vi "Read Write Sample Code - JKI SM.vi"(8 "error in (no error)":errorcluster) -> (0 "error out":errorcluster)   [LabVIEW 2020]
panel:
  in  "stop":bool
  in  "讀取目標字數":i32=1
  in  "Write":bool
  in  "VISA resource name":refnum<visa-resource-name>
  out "read buffer":string
  in  "write buffer":string
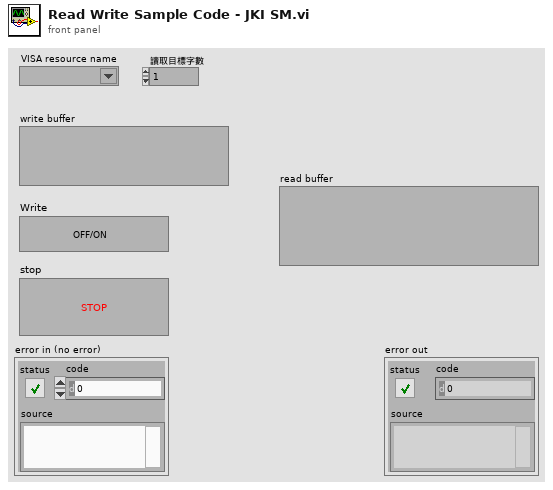
[diagram p1: front panel]
types:
  T1 = enum32{"Invalid", "Standard", "Closed", "Hidden", "Minimized", "Maximized"}
  T2 = enum32{"invalid app kind", "Development System", "Run Time System", "Student Edition", "Embedded LabVIEW", "Evaluation", "Custom"}
  T3 = cluster{"Core":cluster{"Current VI Reference":refnum<vi>, "Close Panel on Exit?":bool}, "VISA resource name":refnum<visa-resource-name>, "Serial Settings:Number of Bytes at Serial Port":u32, "read buffer":string}
  T4 = cluster{"Current VI Reference":refnum<vi>, "Close Panel on Exit?":bool}
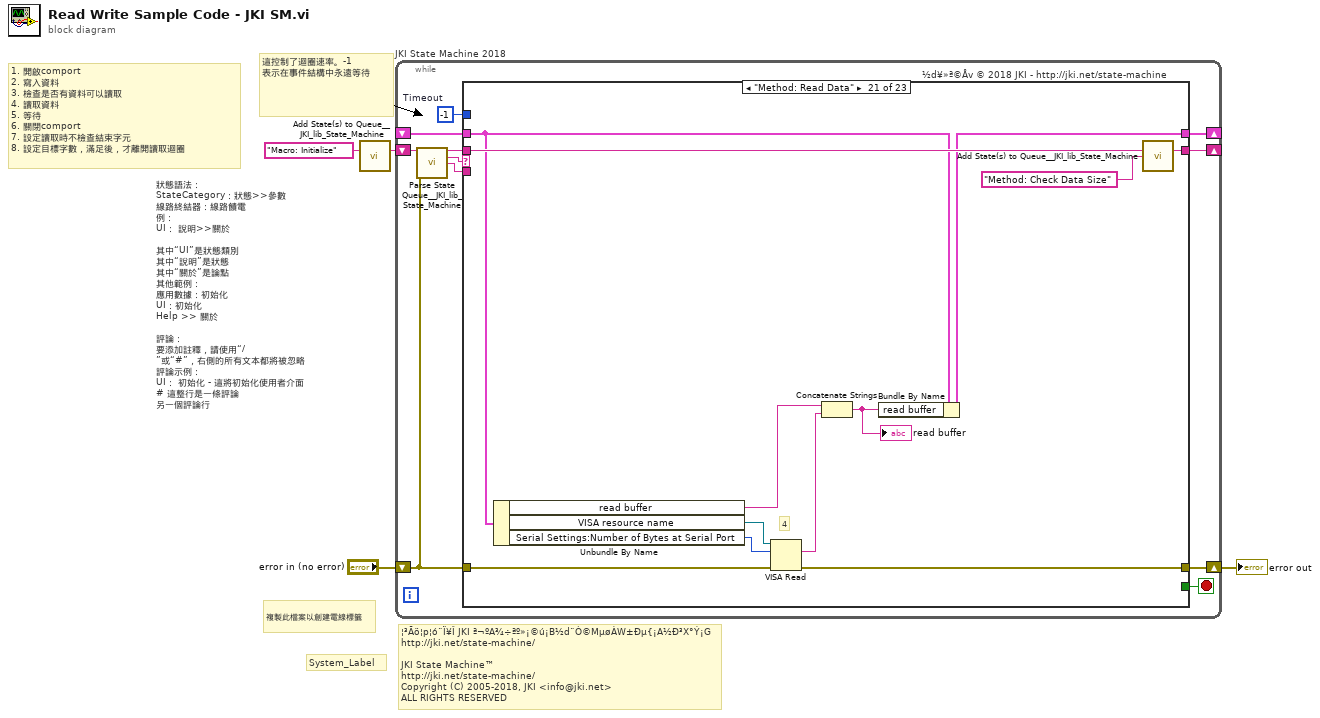
[diagram p0: block diagram]
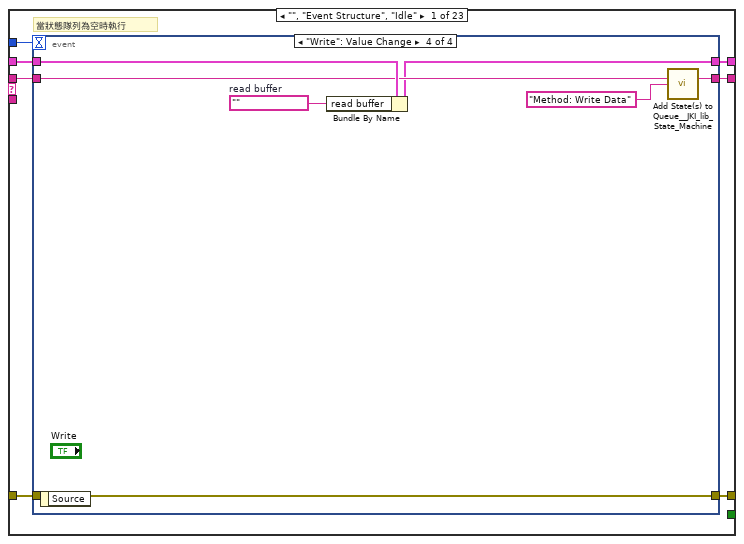
[diagram p2: hidden frame]
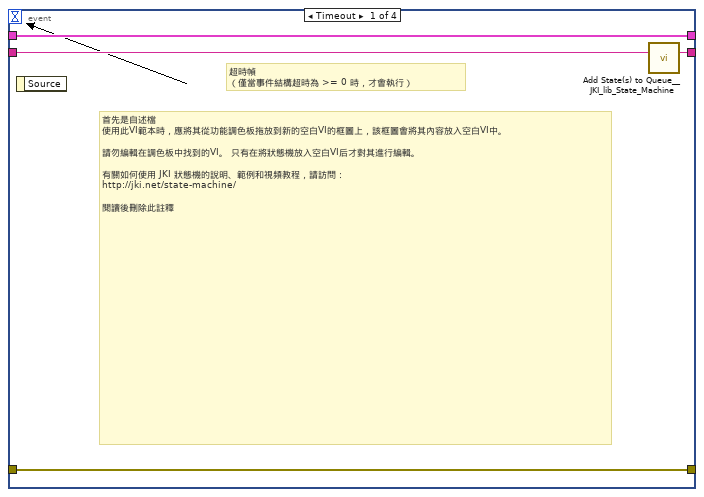
[diagram p3: hidden frame]
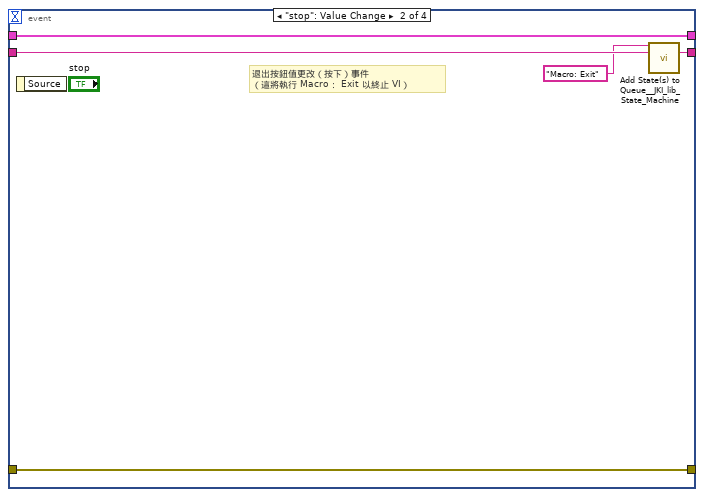
[diagram p4: hidden frame]
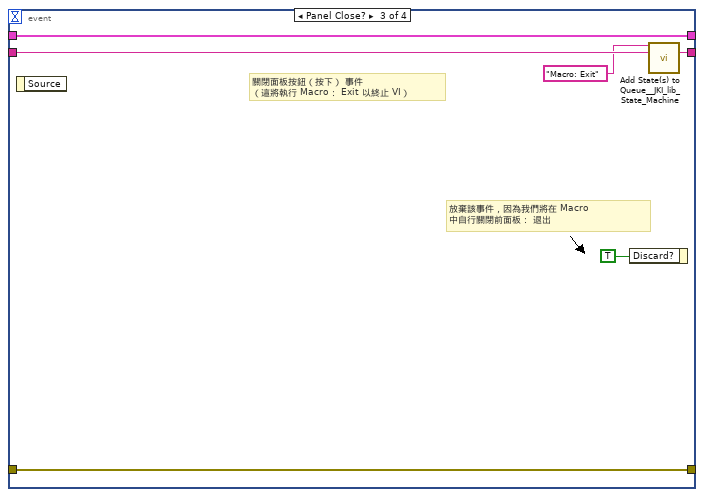
[diagram p5: hidden frame]
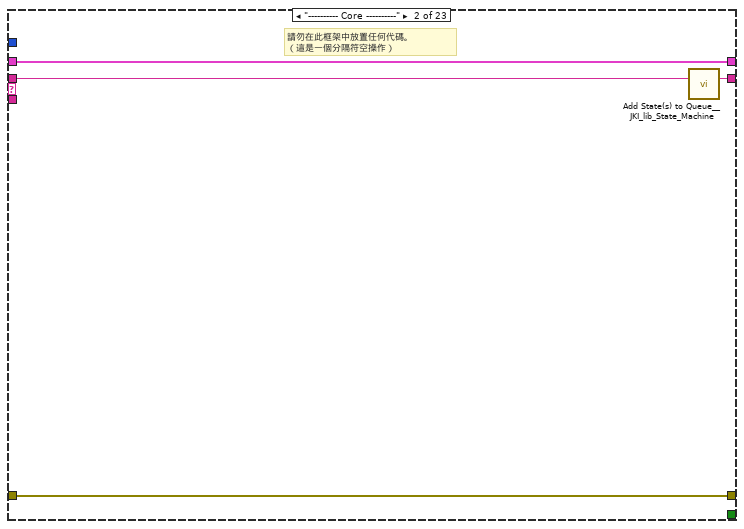
[diagram p6: hidden frame]
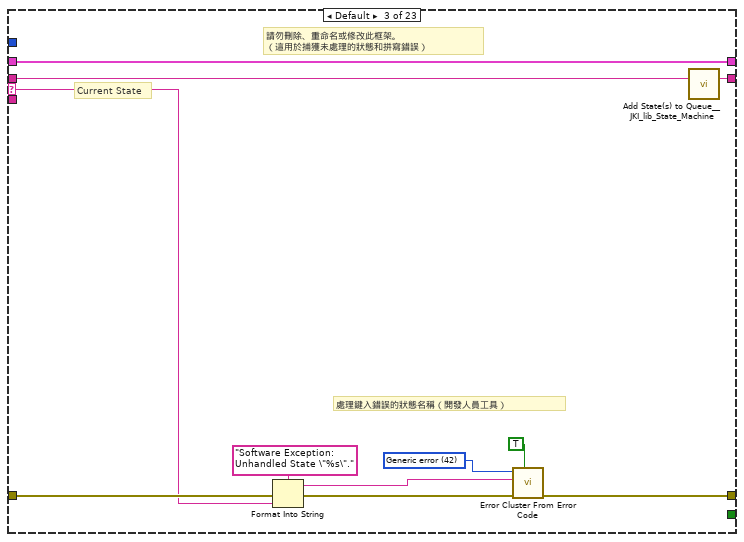
[diagram p7: hidden frame]
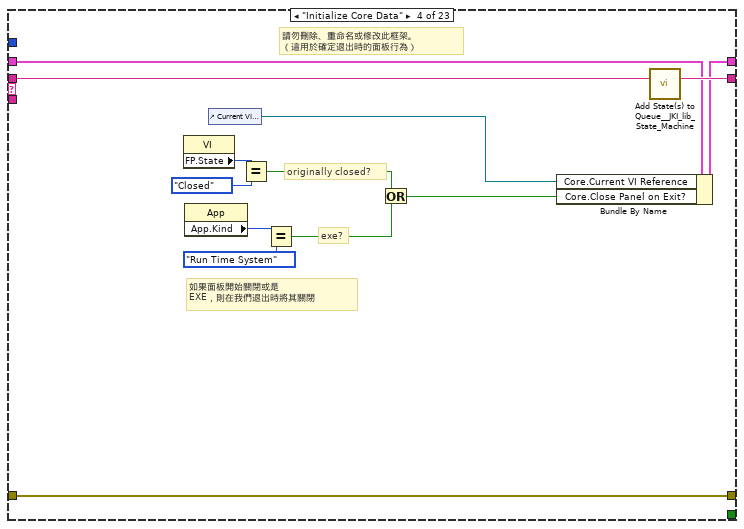
[diagram p8: hidden frame]
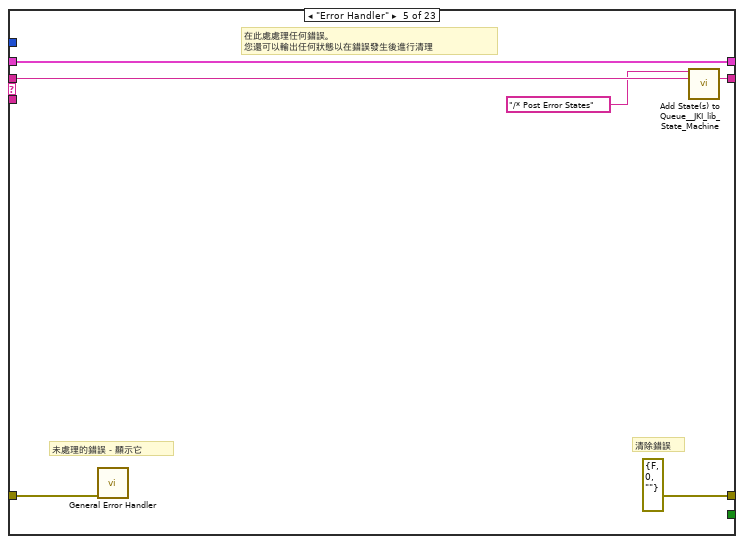
[diagram p9: hidden frame]
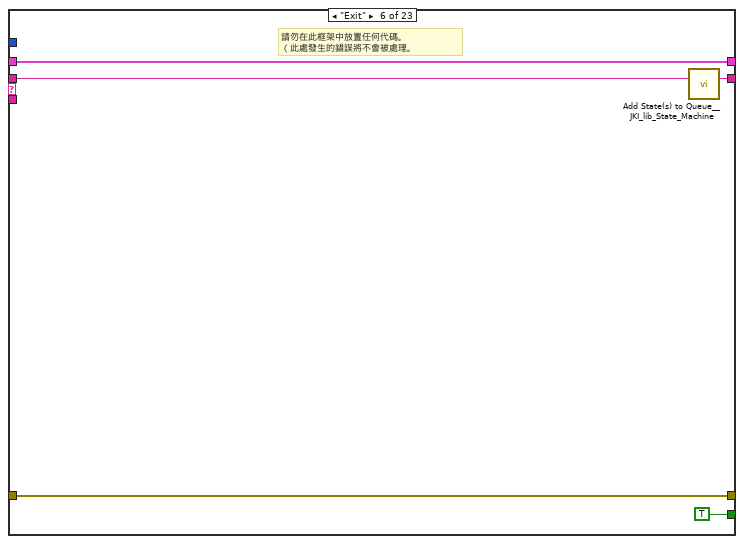
[diagram p10: hidden frame]
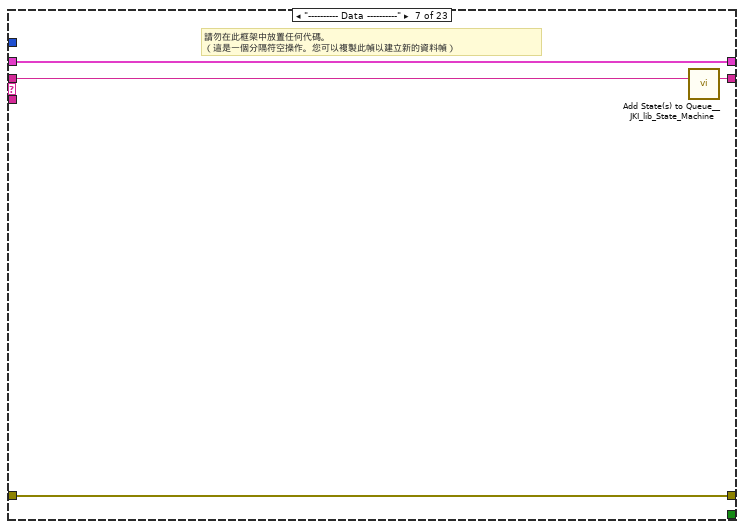
[diagram p11: hidden frame]
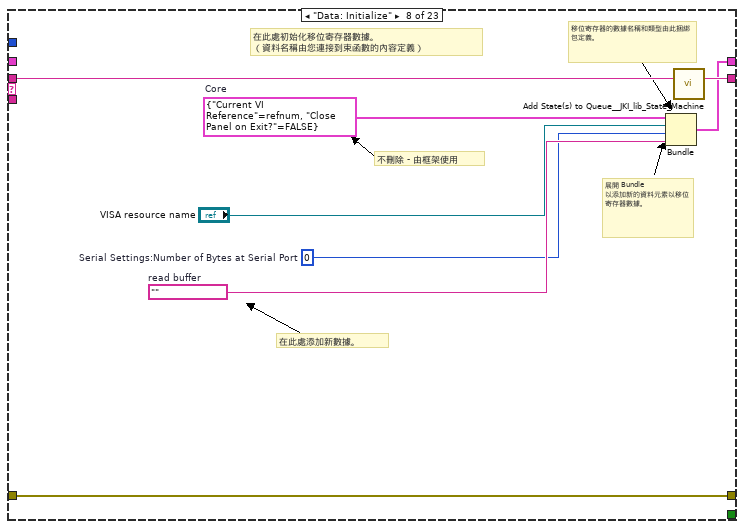
[diagram p12: hidden frame]
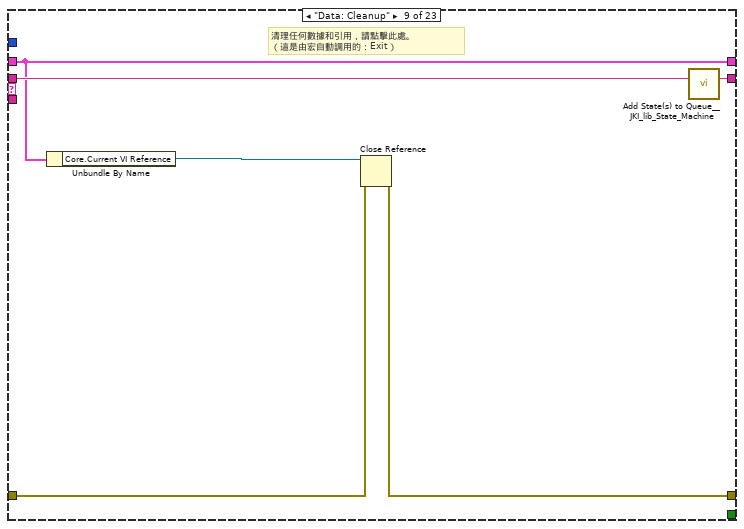
[diagram p13: hidden frame]
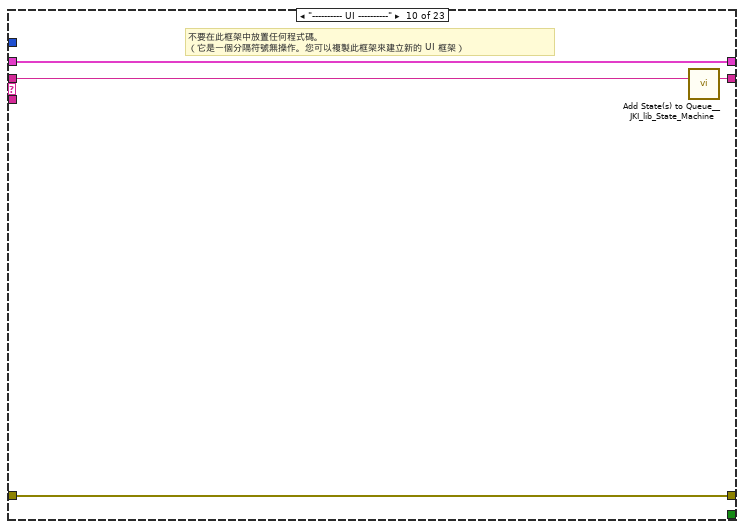
[diagram p14: hidden frame]
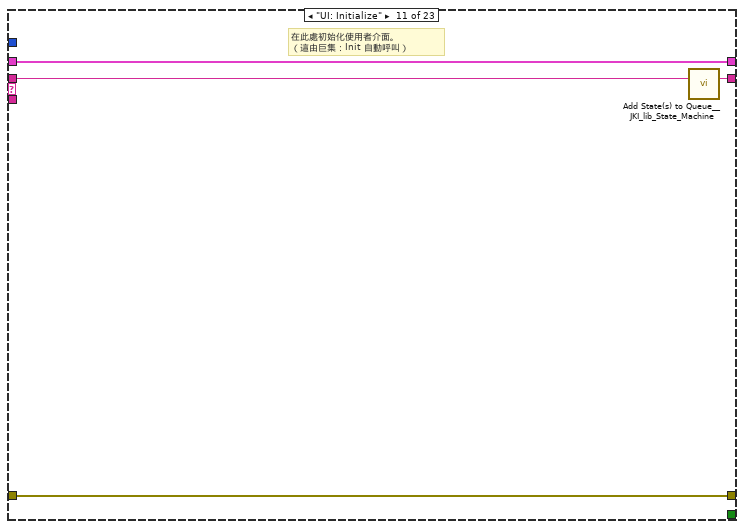
[diagram p15: hidden frame]
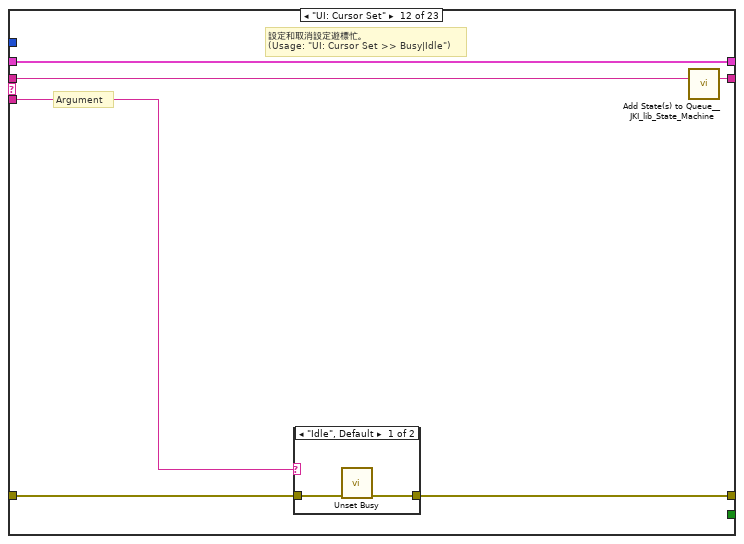
[diagram p16: hidden frame]
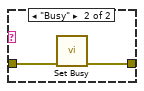
[diagram p17: hidden frame]
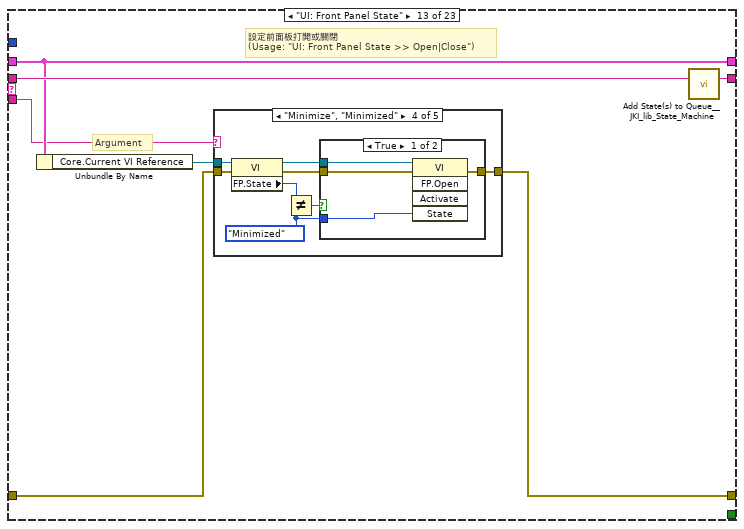
[diagram p18: hidden frame]
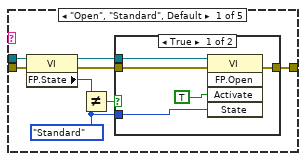
[diagram p19: hidden frame]
diagram:
  # "¦³Ãö¦p¦ó¨Ï¥Î JKI ª¬ºA¾÷ªº»¡©ú¡B½d¨Ò©MµøÀW±Ðµ{¡A½Ð³X°Ý¡G\nhttp://jki.net/state-machine/\n\nJKI State Machine™\nhttp://jki.net/state-machine/\nCopyright (C) 2005-2018, JKI <info@jki.net>\nALL RIGHTS RESERVED"
  # "狀態語法：\nStateCategory：狀態>>參數\n線路終結器：線路饋電\n例：\nUI： 說明>>關於\n\n其中“UI”是狀態類別\n其中“說明”是狀態\n其中“關於”是論點\n其他範例：\n應用數據：初始化\nUI：初始化\nHelp >> 關於\n\n評論：\n要添加註釋，請使用“/”或“#”，右側的所有文本都將被忽略\n評論示例：\nUI： 初始化 - 這將初始化使用者介面\n# 這整行是一條評論\n另一個評論行"
  # "複製此檔案以創建電線標籤"
  # "這控制了迴圈速率。-1 表示在事件結構中永遠等待"
  # "System_Label"
  # "1. 開啟comport\n2. 寫入資料\n3. 檢查是否有資料可以讀取\n4. 讀取資料\n5. 等待\n6. 關閉comport\n7. 設定讀取時不檢查結束字元\n8. 設定目標字數，滿足後，才離開讀取迴圈"
  n1 = call <vilib>:"Add State(s) to Queue__JKI_lib_State_Machine.vi"("State(s) in (\"\")"="Macro: Initialize") -> ("States Out"=w4:string)  [unwired: 14 in]
  n2 = while "JKI State Machine 2018" {
    shift-right: [w8] -> _
    shift-left: _ -> [w7]
    shift-right: [w11] -> w1
    shift-left: "error in (no error)" -> [w5]
    shift-right: [w10] -> _
    shift-left: w4 -> [w12]
    stop <- w9 stop-if-true
    w6 = -1  # Timeout
    # "½d¥»ª©Åv © 2018 JKI - http://jki.net/state-machine"
    n3 = call <vilib>:"Parse State Queue__JKI_lib_State_Machine.vi"("State Queue"=w12, "Error In (no error)"=w5) -> ("Remaining States"=w14:string, "Current State"=w15:string, "Arguments"=w13:string)  [unwired: 11 in]
    n4 = case shown="\"Method: Read Data\"" w15 {
      selector: w15 -> [_ _ w49 _ _ _ _ _ _ _ _ _ _ _ _ _ _ _ _ _ _ _ _]
      tunnel: w14 -> [w22 w48 w53 w72 w78 w83 w87 w95 w101 w105 w109 w115 w126 w195 w200 w210 w214 w220 w233 w241 w253 w264 w272]
      tunnel: w13 -> [_ _ _ _ _ _ _ _ _ _ _ w110 w120 _ _ _ _ _ _ _ _ _ _]
      tunnel: w7 -> [w20 w45 w51 w65 w75 w81 w84 _ w96 w102 w107 w113 w122 w192 w197 w207 w211 w215 w231 w235 w249 w259 w268]
      tunnel: [w19 w46 w55 w69 errorcluster {"status"=FALSE, "code"=0, "source"=""} ("error out") w80 w85 w92 w97 w103 w106 w111 w123 w193 w198 w208 w212 w217 w230 w237 w251 w262 w270] -> w11
      tunnel: w5 -> [w18 w46 w54 w69 w74 w80 w85 w92 w98 w103 w106 w112 w124 w193 w198 w208 w212 w218 w229 w236 w250 w262 w269]
      tunnel: [w21 w47 w52 w71 w77 w82 w86 w94 w100 w104 w108 w114 w125 w194 w199 w209 w213 w219 w232 w240 w252 w263 w271] -> w10
      tunnel: [_ _ _ _ _ TRUE _ _ _ _ _ _ _ _ _ _ _ _ _ _ _ _ _] -> w9
      tunnel: [w17 w45 w51 w70 w75 w81 w84 w93 w96 w102 w107 w113 w122 w192 w197 w207 w211 w216 w231 w235 w246 w259 w268] -> w8
      tunnel: w6 -> [w16 _ _ _ _ _ _ _ _ _ _ _ _ _ _ _ _ _ _ _ _ _ _]
      frame "", "Event Structure", "Idle" {
        # "當狀態隊列為空時執行"
        n5 = event shown="[3] \"Write\": Value Change" {
          selector: _ -> [_ _ _ _]
          dyn-events: _ -> [_ _ _ _]
          timeout: w16 -> [_ _ _ _]
          tunnel: w22 -> [w26 w31 w37 w41]
          tunnel: [w25 w30 w36 w42] -> w21
          tunnel: w20 -> [w23 w28 w34 w44]
          tunnel: [w24 w29 w35 w43] -> w19
          tunnel: w18 -> [w24 w29 w35 w43]
          tunnel: [w23 w28 w34 w40] -> w17
          event Timeout {
            # "首先是自述檔\n使用此VI範本時，應將其從功能調色板拖放到新的空白VI的框圖上，該框圖會將其內容放入空白VI中。\n\n請勿編輯在調色板中找到的VI。 只有在將狀態機放入空白VI后才對其進行編輯。\n\n有關如何使用 JKI 狀態機的說明、範例和視頻教程，請訪問：\nhttp://jki.net/state-machine/\n\n閱讀後刪除此註釋"
            # "超時幀\n（僅當事件結構超時為 >= 0 時，才會執行）"
            n6 = event-data() -> ()  [unwired: 1 in, 1 out]
            n7 = call <vilib>:"Add State(s) to Queue__JKI_lib_State_Machine.vi"("State(s) in (\"\")"=w26) -> ("States Out"=w25:string)  [unwired: 14 in]
          }
          event "stop": Value Change {
            # "退出按鈕值更改（按下）事件\n（這將執行 Macro： Exit 以終止 VI）"
            n8 = event-data() -> ()  [unwired: 1 in, 1 out]
            n9 = call <vilib>:"Add State(s) to Queue__JKI_lib_State_Machine.vi"("State(s) in Front (\"\")"="Macro: Exit", "State(s) in (\"\")"=w31) -> ("States Out"=w30:string)  [unwired: 13 in]
          }
          event Panel Close? {
            # "放棄該事件，因為我們將在 Macro 中自行關閉前面板： 退出"
            # "關閉面板按鈕（按下） 事件\n（這將執行 Macro： Exit 以終止 VI）"
            n10 = event-data() -> ()  [unwired: 1 in, 1 out]
            n11 = event-data("Discard?"=TRUE) -> ()  [unwired: 1 in, 1 out]
            n12 = call <vilib>:"Add State(s) to Queue__JKI_lib_State_Machine.vi"("State(s) in Front (\"\")"="Macro: Exit", "State(s) in (\"\")"=w37) -> ("States Out"=w36:string)  [unwired: 13 in]
          }
          event "Write": Value Change {
            w39 = ""  # read buffer
            n13 = event-data() -> ()  [unwired: 1 in, 1 out]
            n14 = Bundle By Name(cluster=w44, "read buffer"=w39) -> (w40:T3)
            n15 = call <vilib>:"Add State(s) to Queue__JKI_lib_State_Machine.vi"("State(s) in (\"\")"=w41, "State(s) at Back (\"\")"="Method: Write Data" ("State(s) at Back (\"\")")) -> ("States Out"=w42:string)  [unwired: 13 in]
          }
        }
      }
      frame "---------- Core ----------" {
        # "請勿在此框架中放置任何代碼。\n（這是一個分隔符空操作）"
        n16 = call <vilib>:"Add State(s) to Queue__JKI_lib_State_Machine.vi"("State(s) in (\"\")"=w48) -> ("States Out"=w47:string)  [unwired: 14 in]
      }
      frame Default {
        w58 = 42 items=["No error", "Argument error", "Memory is full", "Out of zone", "End of file", "File already open", "Generic file I/O error", "File not found", "File permission error", "Disk is full", "Duplicate path", "Too many files open", "System feature not enabled", "Resource file not found", "Cannot add resource", "Resource not found", "Image not found", "Image memory error", "Pen does not exist", "Config type invalid", "Config token not found", "Config parse error", "Config memory error", "Bad external code format", "Bad external code offset", "External code not present", "Null window", "Destroy window error", "Null menu", "Print aborted", "Bad print record", "Print driver error", "Windows error during printing", "Memory error during printing", "Print dialog error", "Generic print error", "Invalid device refnum", "Device not found", "Device parameter error", "Device unit error", "Cannot open device", "Device call aborted", "Generic error", "Cancelled by user", "Object ID too low", "Object ID too high", "Object not in heap", "Unknown heap", "Unknown object (invalid DefProc)", "Unknown object (DefProc not in table)", "Message out of range", "Invalid (null) method", "Unknown message", "Manager call not supported", "Bad address", "Network operation in progress", "Network operation timed out", "Connection is busy", "Network attribute not supported", "Network error", "Address in use", "System out of memory", "Connection aborted", "Connection refused", "Not connected", "Already connected", "Connection closed", "Initialization error (interapplication manager)", "Bad occurrence", "Wait on unbound occurrence handler", "Occurrence queue overflow", "Datalog type conflict", "Unused", "Unrecognized type (interapplication manager)", "Memory corrupt", "Failed to make temporary DLL", "Old CIN version", "Drag socket not found", "Failed to load drop-object", "Failed to register OLE object", "Failed to release OLE object", "Format specifier type mismatch", "Unknown format specifier", "Too few format specifiers", "Too many format specifiers", "Scan failed", "Newer CIN version", "Error converting to variant", "Runtime menu error", "Password tampered", "Variant attribute not found", "Incompatible variant data type", "Event data is not available", "Event Store is not present", "Occurrence is not found", "Event Queue is not created", "Event info is not available", "Refnum passed is NULL", "Error retrieving Class GUID", "Error retrieving CoClass GUID", "Error retrieving TypeLib GUID.", "Bad built application magic bytes.", "Specific driver is different from the specific driver associated with the Logical Name.", "There is no session opened to the class driver.", "Max Error", "MAX - Error with config objects", "MAX - Error loading configuration", "MAX - Group not supported"]
        # "Current State"
        # "請勿刪除、重命名或修改此框架。\n（這用於捕獲未處理的狀態和拼寫錯誤）"
        # "處理鍵入錯誤的狀態名稱（開發人員工具）"
        n17 = Format Into String(format string="Software Exception: Unhandled State \"%s\"." ("message"), error in=w54, w49) -> (resulting string=w57:string, error out=w56:errorcluster)  [unwired: 1 in]
        n18 = call <vilib>:"Error Cluster From Error Code.vi"("show call chain? (False)"=TRUE, "error in (no error)"=w56, "error message (\"\")"=w57, "error code (0)"=w58) -> ("error out"=w55:errorcluster)  [unwired: 5 in]
        n19 = call <vilib>:"Add State(s) to Queue__JKI_lib_State_Machine.vi"("State(s) in (\"\")"=w53) -> ("States Out"=w52:string)  [unwired: 14 in]
      }
      frame "Initialize Core Data" {
        # "請勿刪除、重命名或修改此框架。\n（這用於確定退出時的面板行為）"
        # "originally closed?"
        # "exe?"
        # "如果面板開始關閉或是 EXE，則在我們退出時將其關閉"
        n20 = property class="VI"() -> ("FP.State"=w62:T1)  [unwired: 2 in, 2 out]
        n21 = property class="App"() -> ("App.Kind"=w68:T2)  [unwired: 2 in, 2 out]
        n22 = control-ref of="Current VI Reference"() -> (w63:refnum<vi>)
        n23 = Equal?(x=w62, y=T1."Closed" ("Front Panel Window:State")) -> (x = y?=w60:bool)
        n24 = Equal?(x=w68, y=T2."Run Time System" ("Application:Kind")) -> (x = y?=w66:bool)
        n25 = Or(x=w60, y=w66) -> (x .or. y?=w64:bool)
        n26 = Bundle By Name(cluster=w65, "Core.Current VI Reference"=w63, "Core.Close Panel on Exit?"=w64) -> (w70:T3)
        n27 = call <vilib>:"Add State(s) to Queue__JKI_lib_State_Machine.vi"("State(s) in (\"\")"=w72) -> ("States Out"=w71:string)  [unwired: 14 in]
      }
      frame "Error Handler" {
        # "未處理的錯誤－顯示它"
        # "在此處處理任何錯誤。\n您還可以輸出任何狀態以在錯誤發生後進行清理"
        # "清除錯誤"
        n28 = call <vilib>:"General Error Handler.vi"("error in (no error)"=w74) -> ()  [unwired: 10 in, 5 out]
        n29 = call <vilib>:"Add State(s) to Queue__JKI_lib_State_Machine.vi"("State(s) in Front (\"\")"="/* Post Error States", "State(s) in (\"\")"=w78) -> ("States Out"=w77:string)  [unwired: 13 in]
      }
      frame "Exit" {
        # "請勿在此框架中放置任何代碼。\n（此處發生的錯誤將不會被處理。"
        n30 = call <vilib>:"Add State(s) to Queue__JKI_lib_State_Machine.vi"("State(s) in (\"\")"=w83) -> ("States Out"=w82:string)  [unwired: 14 in]
      }
      frame "---------- Data ----------" {
        # "請勿在此框架中放置任何代碼。\n（這是一個分隔符空操作。您可以複製此幀以建立新的資料幀）"
        n31 = call <vilib>:"Add State(s) to Queue__JKI_lib_State_Machine.vi"("State(s) in (\"\")"=w87) -> ("States Out"=w86:string)  [unwired: 14 in]
      }
      frame "Data: Initialize" {
        w88 = u32 0  # Serial Settings:Number of Bytes at Serial Port
        w90 = T4 {"Current VI Reference"=refnum, "Close Panel on Exit?"=FALSE}  # Core
        w91 = ""  # read buffer
        # "不刪除 - 由框架使用"
        # "展開 Bundle 以添加新的資料元素以移位寄存器數據。"
        # "在此處添加新數據。"
        # "移位寄存器的數據名稱和類型由此捆綁包定義。"
        # "在此處初始化移位寄存器數據。\n（資料名稱由您連接到束函數的內容定義）"
        n32 = Bundle("Core"=w90, "VISA resource name"="VISA resource name", "Serial Settings:Number of Bytes at Serial Port"=w88, "read buffer"=w91) -> (w93:T3)  [unwired: 1 in]
        n33 = call <vilib>:"Add State(s) to Queue__JKI_lib_State_Machine.vi"("State(s) in (\"\")"=w95) -> ("States Out"=w94:string)  [unwired: 14 in]
      }
      frame "Data: Cleanup" {
        # "清理任何數據和引用，請點擊此處。\n（這是由宏自動調用的：Exit）"
        n34 = Unbundle By Name(w96) -> ("Core.Current VI Reference"=w99:refnum<vi>)
        n35 = Close Reference(reference=w99, error in (no error)=w98) -> (error out=w97:errorcluster)
        n36 = call <vilib>:"Add State(s) to Queue__JKI_lib_State_Machine.vi"("State(s) in (\"\")"=w101) -> ("States Out"=w100:string)  [unwired: 14 in]
      }
      frame "---------- UI ----------" {
        # "不要在此框架中放置任何程式碼。\n（它是一個分隔符號無操作。您可以複製此框架來建立新的 UI 框架）"
        n37 = call <vilib>:"Add State(s) to Queue__JKI_lib_State_Machine.vi"("State(s) in (\"\")"=w105) -> ("States Out"=w104:string)  [unwired: 14 in]
      }
      frame "UI: Initialize" {
        # "在此處初始化使用者介面。\n（這由巨集：Init 自動呼叫）"
        n38 = call <vilib>:"Add State(s) to Queue__JKI_lib_State_Machine.vi"("State(s) in (\"\")"=w109) -> ("States Out"=w108:string)  [unwired: 14 in]
      }
      frame "UI: Cursor Set" {
        # "Argument"
        # "設定和取消設定遊標忙。\n(Usage: \"UI: Cursor Set >> Busy|Idle\")"
        n39 = case shown="\"Idle\", Default" w110 {
          tunnel: w112 -> [w117 w119]
          tunnel: [w116 w118] -> w111
          frame "Idle", Default {
            n40 = call <vilib>:"Unset Busy.vi"("error in (no error)"=w117) -> ("error out"=w116:errorcluster)  [unwired: 10 in]
          }
          frame "Busy" {
            n41 = call <vilib>:"Set Busy.vi"("error in (no error)"=w119) -> ("error out"=w118:errorcluster)  [unwired: 9 in, 1 out]
          }
        }
        n42 = call <vilib>:"Add State(s) to Queue__JKI_lib_State_Machine.vi"("State(s) in (\"\")"=w115) -> ("States Out"=w114:string)  [unwired: 14 in]
      }
      frame "UI: Front Panel State" {
        # "Argument"
        # "設定前面板打開或關閉\n(Usage: \"UI: Front Panel State >> Open|Close\")"
        n43 = Unbundle By Name(w122) -> ("Core.Current VI Reference"=w121:refnum<vi>)
        n44 = case shown="\"Minimize\", \"Minimized\"" w120 {
          tunnel: w124 -> [w132 w147 w158 w171 w184]
          tunnel: [w134 w148 w160 w173 w186] -> w123
          tunnel: w121 -> [w133 w145 w159 w172 w185]
          frame "Open", "Standard", Default {
            w127 = T1."Standard" ("State")
            n45 = property class="VI"(reference=w133, error in=w132) -> (reference out=w130:refnum<vi>, error out=w131:errorcluster, "FP.State"=w129:T1)
            n46 = Not Equal?(x=w129, y=w127) -> (x != y?=w128:bool)
            n47 = case shown="True" w128 {
              tunnel: [w138 w140] -> w134
              tunnel: w131 -> [w137 w140]
              tunnel: w130 -> [w136 _]
              tunnel: w127 -> [w135 _]
              frame True {
                n48 = invoke class="VI" method="FP.Open"(reference=w136, error in=w137, "Activate"=TRUE, "State"=w135) -> (error out=w138:errorcluster)  [unwired: 1 in, 4 out]
              }
              frame False {
              }
            }
          }
          frame "Close", "Closed" {
            n49 = property class="VI"(reference=w145, error in=w147) -> (reference out=w144:refnum<vi>, error out=w146:errorcluster, "FP.State"=w142:T1)
            n50 = Not Equal?(x=w142, y=T1."Closed" ("Front Panel Window:State")) -> (x != y?=w141:bool)
            n51 = case shown="True" w141 {
              tunnel: [w149 w152] -> w148
              tunnel: w146 -> [w149 w151]
              tunnel: w144 -> [_ w150]
              frame False {
              }
              frame True {
                n52 = invoke class="VI" method="FP.Close"(reference=w150, error in=w151) -> (error out=w152:errorcluster)  [unwired: 1 in, 2 out]
              }
            }
          }
          frame "Hidden", "Hide" {
            w153 = T1."Hidden" ("State")
            n53 = property class="VI"(reference=w159, error in=w158) -> (reference out=w156:refnum<vi>, error out=w157:errorcluster, "FP.State"=w155:T1)
            n54 = Not Equal?(x=w155, y=w153) -> (x != y?=w154:bool)
            n55 = case shown="True" w154 {
              tunnel: [w164 w165] -> w160
              tunnel: w157 -> [w163 w165]
              tunnel: w156 -> [w162 _]
              tunnel: w153 -> [w161 _]
              frame True {
                n56 = invoke class="VI" method="FP.Open"(reference=w162, error in=w163, "State"=w161) -> (error out=w164:errorcluster)  [unwired: 2 in, 4 out]
              }
              frame False {
              }
            }
          }
          frame "Minimize", "Minimized" {
            w166 = T1."Minimized" ("State")
            n57 = property class="VI"(reference=w172, error in=w171) -> (reference out=w169:refnum<vi>, error out=w170:errorcluster, "FP.State"=w168:T1)
            n58 = Not Equal?(x=w168, y=w166) -> (x != y?=w167:bool)
            n59 = case shown="True" w167 {
              tunnel: [w177 w178] -> w173
              tunnel: w170 -> [w176 w178]
              tunnel: w169 -> [w175 _]
              tunnel: w166 -> [w174 _]
              frame True {
                n60 = invoke class="VI" method="FP.Open"(reference=w175, error in=w176, "State"=w174) -> (error out=w177:errorcluster)  [unwired: 2 in, 4 out]
              }
              frame False {
              }
            }
          }
          frame "Maximize", "Maximized" {
            w179 = T1."Maximized" ("State")
            n61 = property class="VI"(reference=w185, error in=w184) -> (reference out=w182:refnum<vi>, error out=w183:errorcluster, "FP.State"=w181:T1)
            n62 = Not Equal?(x=w181, y=w179) -> (x != y?=w180:bool)
            n63 = case shown="True" w180 {
              tunnel: [w190 w191] -> w186
              tunnel: w183 -> [w189 w191]
              tunnel: w182 -> [w188 _]
              tunnel: w179 -> [w187 _]
              frame True {
                n64 = invoke class="VI" method="FP.Open"(reference=w188, error in=w189, "State"=w187) -> (error out=w190:errorcluster)  [unwired: 2 in, 4 out]
              }
              frame False {
              }
            }
          }
        }
        n65 = call <vilib>:"Add State(s) to Queue__JKI_lib_State_Machine.vi"("State(s) in (\"\")"=w126) -> ("States Out"=w125:string)  [unwired: 14 in]
      }
      frame "---------- Macro ----------" {
        # "不要在此框架中放置任何程式碼。\n（它是一個分隔符無操作。您可以複製該幀以創建新的巨集幀）"
        n66 = call <vilib>:"Add State(s) to Queue__JKI_lib_State_Machine.vi"("State(s) in (\"\")"=w195) -> ("States Out"=w194:string)  [unwired: 14 in]
      }
      frame "Macro: Initialize" {
        w196 = "Data: Initialize\nInitialize Core Data\nUI: Initialize\nUI: Front Panel State >> Open"  # Data: Initialize Initialize Core Data UI: Initialize UI: Front Panel State >> Open
        # "初始化巨集\n（當VI啟動時調用一次）"
        n67 = call <vilib>:"Add State(s) to Queue__JKI_lib_State_Machine.vi"("State(s) in Front (\"\")"=w196, "State(s) in (\"\")"=w200) -> ("States Out"=w199:string)  [unwired: 13 in]
      }
      frame "Macro: Exit" {
        # "退出宏\n（當VI退出時調用一次）"
        n68 = Unbundle By Name(w207) -> ("Core.Close Panel on Exit?"=w206:bool)
        n69 = Select(t="UI: Front Panel State >> Close", s=w206, f="") -> (s? t:f=w203:string)
        n70 = call <vilib>:"Add State(s) to Queue__JKI_lib_State_Machine.vi"("State(s) in (\"\")"=w203, "State(s) at Back (\"\")"="Data: Cleanup\nExit") -> ("States Out"=w201:string)  [unwired: 13 in]
        n71 = call <vilib>:"Add State(s) to Queue__JKI_lib_State_Machine.vi"("State(s) in Front (\"\")"=w201, "State(s) in (\"\")"=w210) -> ("States Out"=w209:string)  [unwired: 13 in]
      }
      frame "---------- Method ----------" {
        # "模板分隔符\n（您可以複製或修改此框架）"
        n72 = call <vilib>:"Add State(s) to Queue__JKI_lib_State_Machine.vi"("State(s) in (\"\")"=w214) -> ("States Out"=w213:string)  [unwired: 14 in]
      }
      frame "Method: Open Port" {
        n73 = in-place {
          in-place-border: w218 -> [w224]
          in-place-border: [w223] -> w217
          w225 = u16 0 items=["None", "Last Bit", "TermChar"] ("Serial Settings:End Mode for Reads")
          # "7"
          # "1"
          n74 = in-place-cluster #1(w215) -> ("VISA resource name"=w222:refnum<visa-resource-name>)
          n75 = VISA Open(error in (no error)=w224, VISA resource name=w222) -> (VISA resource name=w227:refnum<visa-resource-name>, error out=w226:errorcluster)  [unwired: 3 in]
          n76 = property class="Instr"(reference=w227, error in=w226, "ASRL End In"=w225) -> (reference out=w221:refnum<visa-resource-name>, error out=w223:errorcluster)
          n77 = in-place-cluster #1("VISA resource name"=w221) -> (w216:T3)
        }
        n78 = call <vilib>:"Add State(s) to Queue__JKI_lib_State_Machine.vi"("State(s) in (\"\")"=w220) -> ("States Out"=w219:string)  [unwired: 14 in]
      }
      frame "Method: Close Port" {
        # "6"
        n79 = Unbundle By Name(w231) -> ("VISA resource name"=w228:refnum<visa-resource-name>)
        n80 = VISA Close(VISA resource name=w228, error in (no error)=w229) -> (error out=w230:errorcluster)
        n81 = call <vilib>:"Add State(s) to Queue__JKI_lib_State_Machine.vi"("State(s) in (\"\")"=w233) -> ("States Out"=w232:string)  [unwired: 14 in]
      }
      frame "Method: Write Data" {
        # "2"
        n82 = Unbundle By Name(w235) -> ("VISA resource name"=w234:refnum<visa-resource-name>)
        n83 = VISA Write(VISA resource name=w234, write buffer="write buffer", error in (no error)=w236) -> (error out=w237:errorcluster)  [unwired: 2 out]
        n84 = call <vilib>:"Add State(s) to Queue__JKI_lib_State_Machine.vi"("State(s) in (\"\")"=w241, "State(s) at Back (\"\")"="Method: Check Data Buffer" ("State(s) at Back (\"\")")) -> ("States Out"=w240:string)  [unwired: 13 in]
      }
      frame "Method: Read Data" {
        # "4"
        n85 = Unbundle By Name(w249) -> ("read buffer"=w245:string, "VISA resource name"=w248:refnum<visa-resource-name>, "Serial Settings:Number of Bytes at Serial Port"=w247:u32)
        n86 = VISA Read(VISA resource name=w248, byte count=w247, error in (no error)=w250) -> (read buffer=w244:string, error out=w251:errorcluster)  [unwired: 2 out]
        n87 = Concatenate Strings(w245, w244) -> (w243:string)
        "read buffer" <- w243
        n88 = Bundle By Name(cluster=w249, "read buffer"=w243) -> (w246:T3)
        n89 = call <vilib>:"Add State(s) to Queue__JKI_lib_State_Machine.vi"("State(s) in (\"\")"=w253, "State(s) at Back (\"\")"="Method: Check Data Size" ("State(s) at Back (\"\")")) -> ("States Out"=w252:string)  [unwired: 13 in]
      }
      frame "Method: Check Data Size" {
        # "8"
        n90 = Unbundle By Name(w259) -> ("read buffer"=w258:string)
        n91 = String Length(string=w258) -> (length=w260:i32)
        n92 = Greater Or Equal?(x=w260, y="讀取目標字數") -> (x >= y?=w257:bool)
        n93 = Select(t="", s=w257, f="Method: Check Data Buffer" ("State(s) at Back (\"\")")) -> (s? t:f=w255:string)
        n94 = call <vilib>:"Add State(s) to Queue__JKI_lib_State_Machine.vi"("State(s) in (\"\")"=w264, "State(s) at Back (\"\")"=w255) -> ("States Out"=w263:string)  [unwired: 13 in]
      }
      frame "Method: Check Data Buffer" {
        # "3"
        n95 = Unbundle By Name(w268) -> ("VISA resource name"=w267:refnum<visa-resource-name>)
        n96 = property class="Instr"(reference=w267, error in=w269) -> (error out=w270:errorcluster, "Bytes at Port"=w266:u32)  [unwired: 1 out]
        n97 = case shown="0, Default" w266 {
          tunnel: [_ "Method: Read Data" ("State(s) at Back (\"\")")] -> w265
          frame 0, Default {
            # "5"
            n98 = Wait (ms)(milliseconds to wait=u32 200) -> ()  [unwired: 1 out]
          }
          frame 1.. {
          }
        }
        n99 = call <vilib>:"Add State(s) to Queue__JKI_lib_State_Machine.vi"("State(s) in (\"\")"=w272, "State(s) at Back (\"\")"=w265) -> ("States Out"=w271:string)  [unwired: 13 in]
      }
    }
  }
  "error out" <- w1
